vi "수업2.vi"() -> ()   [LabVIEW 2014]
panel:
  out "숫자형 2":i32
  out "숫자형":dbl
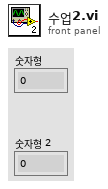
[diagram p1: front panel]
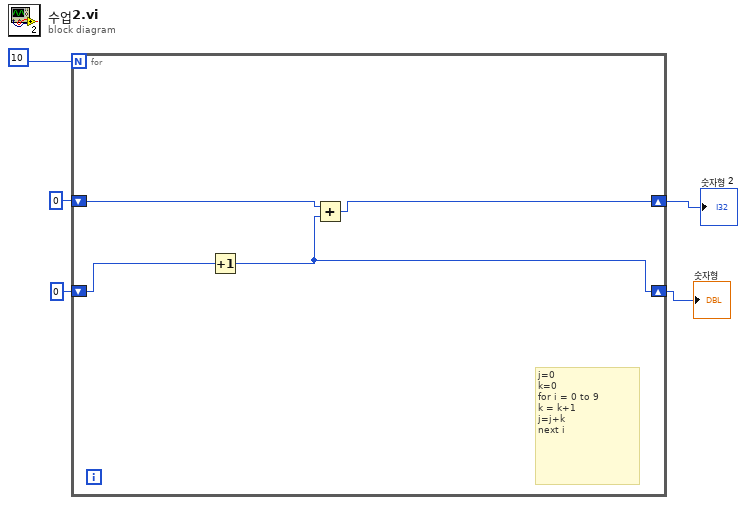
[diagram p0: block diagram]
diagram:
  n1 = for {
    N: 10 -> [_]
    shift-right: [w6] -> w2
    shift-left: 0 -> [w9]
    shift-right: [w8] -> w1
    shift-left: 0 -> [w7]
    # "j=0\nk=0\nfor i = 0 to 9\nk = k+1\nj=j+k\nnext i"
    n2 = Increment(x=w9) -> (x+1=w6:i32)
    n3 = Add(x=w7, y=w6) -> (x+y=w8:i32)
  }
  "숫자형" <- w2
  "숫자형 2" <- w1
